vi "logCtrlWP.vi"(0 "wpPath":path, 1 "time":dbl, 2 "eta_i":dbl[](array[numeric]), 3 "eta_r":dbl[](array[numeric]), 4 "e_i":dbl, 5 "e_psi":dbl, 7 "psiplot":cluster{"psi_d":dbl, "psi":dbl}, 9 "delta":dbl) -> ()   [LabVIEW 2014]
uses:
  <vilib>/Utility/file.llb/Write To Spreadsheet File (DBL).vi
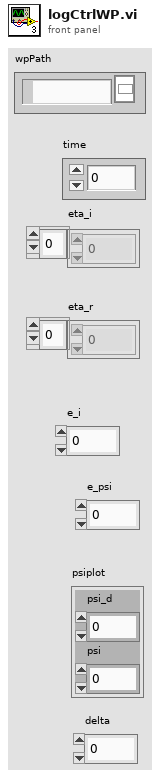
[diagram p1: front panel]
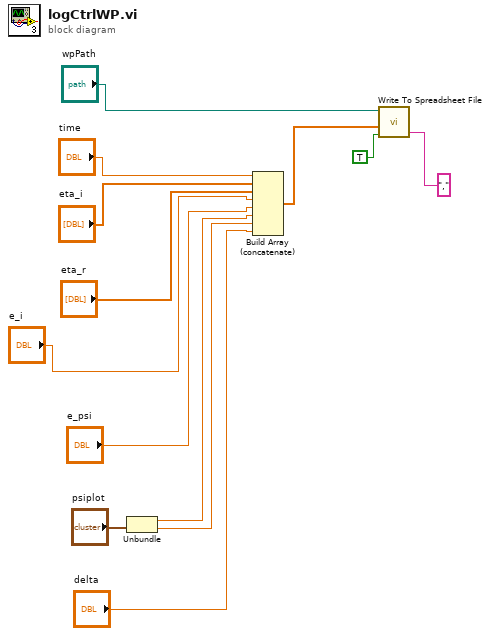
[diagram p0: block diagram]
diagram:
  n1 = Unbundle("psiplot") -> ("psi_d"=w3:dbl, "psi"=w2:dbl)
  n2 = Build Array (concatenate)("time", "eta_i", "eta_r", "e_i", "e_psi", w3, w2, "delta") -> (w13:dbl[])
  n3 = call-poly <vilib>:"Write To Spreadsheet File.vi"("delimiter (\\t)"="," ("delimiter (\\t)"), "append to file? (new file:F)"=TRUE, "1D data"=w13, "file path (dialog if empty)"="wpPath") -> ()  [unwired: 4 in, 1 out]
